vi "FinalizeHWI.vi"(8 "error in (no error)":errorcluster, 10 "Master Device in":refnum<class "Master Device.lvclass">, 11 "Novatech in":refnum<class "Novatech.lvclass">) -> (0 "error out":errorcluster, 2 "Master Device out":refnum<class "Master Device.lvclass">, 3 "Novatech out":refnum<class "Novatech.lvclass">)   [LabVIEW 2013, in "Novatech.lvclass"]
uses:
  Novatech.lvclass
  Master Device/Master Device.lvclass
  Novatech.lvclass/Novatech.ctl
  Novatech 409A.lvlib
panel:
  out "ch2/3 changes?":bool
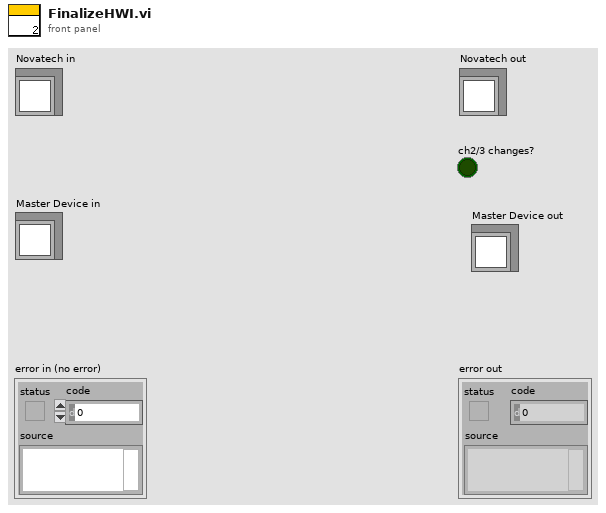
[diagram p1: front panel]
types:
  T1 = cluster{"Triggering":bool[][], "Ramp Info":cluster{"Ramp Index":i32, "Ramp Time":dbl, "Number of Steps":i32}[], "VLIW Array":cluster{"Output Bits":u32, "Data Field":u32, "OP Code":u8, "Delay Count":u64}[]}
  T2 = cluster{"Nova Update List":dbl[][], "2 Freq. [MHz]":dbl, "2 Power [dBm]":u16, "2 phase":u16, "3 Freq. [MHz]":dbl, "3 Power [dBm]":u16, "3 phase":u16}[]
  T3 = cluster{"Freq. [MHz]":dbl[][], "Power [Level]":u16[][], "Phase":u16[][], "2 Freq. [MHz]":dbl, "2 Power [dBm]":u16, "2 phase":u16, "3 Freq. [MHz]":dbl, "3 Power [dBm]":u16, "3 phase":u16}
  T4 = cluster{"Nova Update List":dbl[][], "2 Freq. [MHz]":dbl, "2 Power [dBm]":u16, "2 phase":u16, "3 Freq. [MHz]":dbl, "3 Power [dBm]":u16, "3 phase":u16}
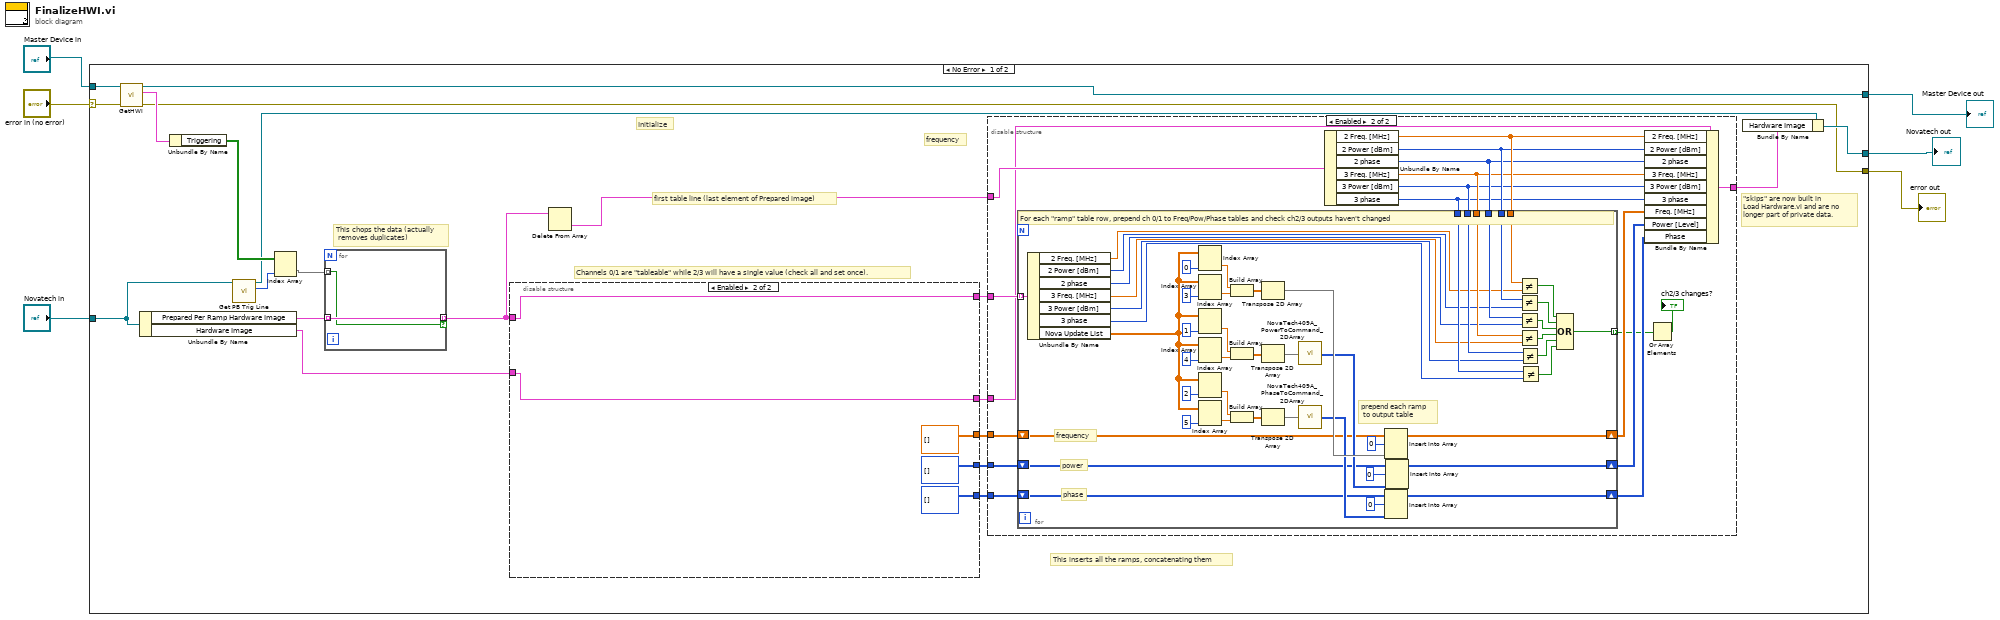
[diagram p0: block diagram]
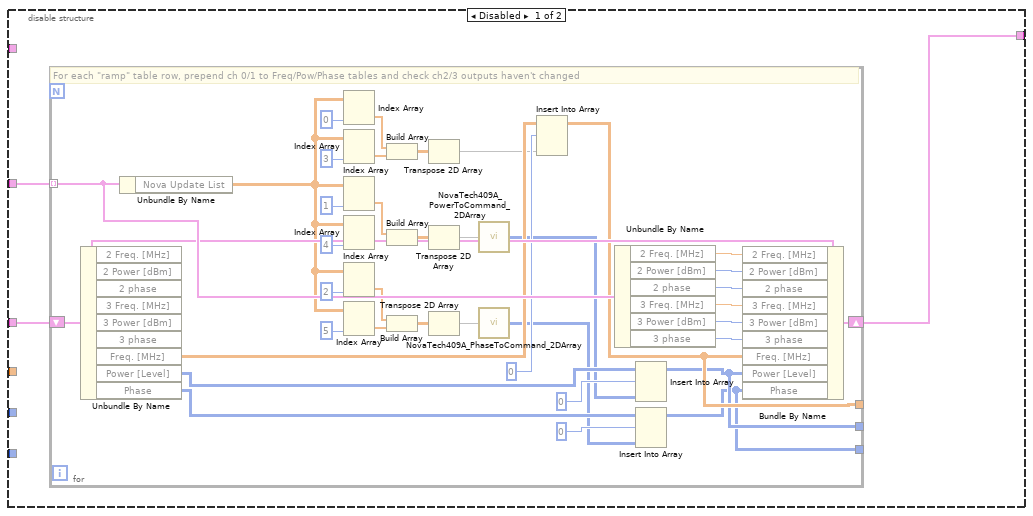
[diagram p2: hidden frame]
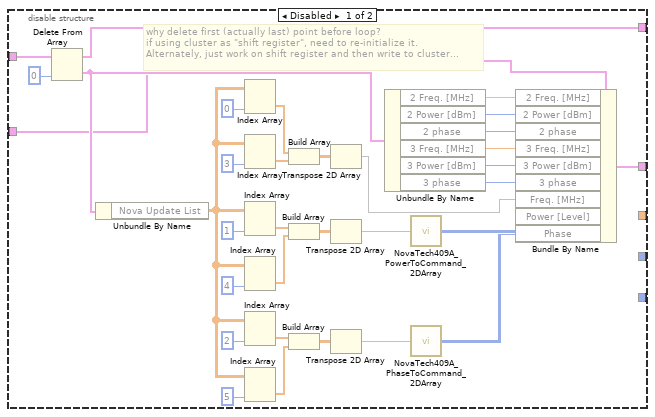
[diagram p3: hidden frame]
diagram:
  n1 = case shown="No Error" "error in (no error)" {
    selector: "error in (no error)" -> [w22 w181]
    tunnel: "Novatech in" -> [w23 w183]
    tunnel: "Master Device in" -> [w26 w182]
    tunnel: [w25 w182] -> w2
    tunnel: [w10 w183] -> w3
    tunnel: [w9 w181] -> w1
    frame No Error {
      # "first table line (last element of Prepared image)"
      # "\"skips\" are now built in \nLoad Hardware.vi and are no \nlonger part of private data."
      # "frequency"
      # "Initialize"
      # "Channels 0/1 are \"tableable\" while 2/3 will have a single value (check all and set once)."
      # "This inserts all the ramps, concatenating them"
      # "This chops the data (actually\n removes duplicates)"
      n2 = call-dynamic "GetHWI.vi"("error in (no error)"=w22, "Master Device in"=w26) -> ("error out"=w9:errorcluster, "Hardware Image"=w24:T1, "Master Device out"=w25:refnum<class "Master Device.lvclass">)  [unwired: 7 in]
      n3 = Unbundle By Name(w23) -> ("Prepared Per Ramp Hardware Image"=w27:T2, "Hardware Image"=w12:T3)
      n4 = Unbundle By Name(w24) -> ("Triggering"=w21:bool[][])
      n5 = call-dynamic "Get PB Trig Line.vi"("Device in"=w23) -> ("PB Trigger Line"=w20:u16, "Device out"=w11:refnum<class "Novatech.lvclass">)  [unwired: 8 in, 1 out]
      n6 = Index Array(array=w21, index (col)=w20) -> (element=w19:bool[])  [unwired: 1 in]
      n7 = for {
        tunnel: w27 -> [w180] mode=indexing
        tunnel: w19 -> [w179] mode=indexing
        tunnel: [w180] -> w8 mode=indexing if=w179
      }
      n8 = disable-structure shown="Enabled" {
        disable-tunnel: w8 -> [w147 w178]
        disable-tunnel: [w144 w177] -> w17
        disable-tunnel: [w143 w178] -> w16
        disable-tunnel: w12 -> [w141 w177]
        disable-tunnel: [_ dbl[][] [] ("Freq. [MHz]")] -> w15
        disable-tunnel: [_ u16[][] [] ("Power [Level]")] -> w14
        disable-tunnel: [_ u16[][] [] ("Phase")] -> w13
        frame Disabled {
          # "why delete first (actually last) point before loop?\nif using cluster as \"shift register\", need to re-initialize it.\nAlternately, just work on shift register and then write to cluster..."
          n9 = Delete From Array(array=w147, index=0) -> (deleted portion=w145:T4, array with subset deleted=w143:T2)  [unwired: 1 in]
          n10 = Unbundle By Name(w145) -> ("Nova Update List"=w155:dbl[][])
          n11 = Index Array(array=w155, index (col)=0) -> (element=w165:dbl[])  [unwired: 1 in]
          n12 = Index Array(array=w155, index (col)=3) -> (element=w164:dbl[])  [unwired: 1 in]
          n13 = Index Array(array=w155, index (col)=1) -> (element=w161:dbl[])  [unwired: 1 in]
          n14 = Index Array(array=w155, index (col)=4) -> (element=w160:dbl[])  [unwired: 1 in]
          n15 = Index Array(array=w155, index (col)=2) -> (element=w157:dbl[])  [unwired: 1 in]
          n16 = Index Array(array=w155, index (col)=5) -> (element=w156:dbl[])  [unwired: 1 in]
          n17 = Build Array(w165, w164) -> (w154:dbl[][])
          n18 = Build Array(w161, w160) -> (w153:dbl[][])
          n19 = Build Array(w157, w156) -> (w152:dbl[][])
          n20 = Transpose 2D Array(2D array=w154) -> (transposed array=w151:dbl[][])
          n21 = Transpose 2D Array(2D array=w153) -> (transposed array=w150:dbl[][])
          n22 = Transpose 2D Array(2D array=w152) -> (transposed array=w148:dbl[][])
          n23 = Unbundle By Name(w145) -> ("2 Freq. [MHz]"=w173:dbl, "2 Power [dBm]"=w172:u16, "2 phase"=w171:u16, "3 Freq. [MHz]"=w170:dbl, "3 Power [dBm]"=w169:u16, "3 phase"=w168:u16)
          n24 = call "NovaTech409A_PowerToCommand_2DArray.vi"("Novatech Power [dBm]"=w150) -> ("Novatech Command"=w149:u16[][])
          n25 = call "NovaTech409A_PhaseToCommand_2DArray.vi"("Novatech Phase [degrees]"=w148) -> ("Novatech Command"=w142:u16[][])
          n26 = Bundle By Name(cluster=w141, "2 Freq. [MHz]"=w173, "2 Power [dBm]"=w172, "2 phase"=w171, "3 Freq. [MHz]"=w170, "3 Power [dBm]"=w169, "3 phase"=w168, "Freq. [MHz]"=w151, "Power [Level]"=w149, "Phase"=w142) -> (w144:T3)
        }
        frame Enabled {
        }
      }
      n27 = Delete From Array(array=w8) -> (deleted portion=w7:T4)  [unwired: 2 in, 1 out]
      n28 = disable-structure shown="Enabled" {
        disable-tunnel: [w33 w86] -> w18
        disable-tunnel: w17 -> [w32 w73]
        disable-tunnel: w16 -> [w31 w90]
        disable-tunnel: w15 -> [_ w89]
        disable-tunnel: w14 -> [_ w88]
        disable-tunnel: w13 -> [_ w87]
        disable-tunnel: w7 -> [_ w82]
        frame Disabled {
          n29 = for {
            tunnel: w31 -> [w72] mode=indexing
            shift-right: [w70] -> w33
            shift-left: w32 -> [w71]
            tunnel: [w69] -> w30
            tunnel: [w68] -> w29
            tunnel: [w34] -> w28
            # "For each \"ramp\" table row, prepend ch 0/1 to Freq/Pow/Phase tables and check ch2/3 outputs haven't changed"
            n30 = Unbundle By Name(w71) -> ("Freq. [MHz]"=w47:dbl[][], "Power [Level]"=w41:u16[][], "Phase"=w40:u16[][])  [unwired: 6 out]
            n31 = Unbundle By Name(w72) -> ("Nova Update List"=w48:dbl[][])
            n32 = Index Array(array=w48, index (col)=0) -> (element=w58:dbl[])  [unwired: 1 in]
            n33 = Index Array(array=w48, index (col)=3) -> (element=w57:dbl[])  [unwired: 1 in]
            n34 = Index Array(array=w48, index (col)=1) -> (element=w54:dbl[])  [unwired: 1 in]
            n35 = Index Array(array=w48, index (col)=4) -> (element=w53:dbl[])  [unwired: 1 in]
            n36 = Index Array(array=w48, index (col)=2) -> (element=w50:dbl[])  [unwired: 1 in]
            n37 = Index Array(array=w48, index (col)=5) -> (element=w49:dbl[])  [unwired: 1 in]
            n38 = Build Array(w58, w57) -> (w46:dbl[][])
            n39 = Build Array(w54, w53) -> (w43:dbl[][])
            n40 = Build Array(w50, w49) -> (w42:dbl[][])
            n41 = Transpose 2D Array(2D array=w46) -> (transposed array=w39:dbl[][])
            n42 = Transpose 2D Array(2D array=w43) -> (transposed array=w38:dbl[][])
            n43 = Transpose 2D Array(2D array=w42) -> (transposed array=w36:dbl[][])
            n44 = call "NovaTech409A_PowerToCommand_2DArray.vi"("Novatech Power [dBm]"=w38) -> ("Novatech Command"=w37:u16[][])
            n45 = call "NovaTech409A_PhaseToCommand_2DArray.vi"("Novatech Phase [degrees]"=w36) -> ("Novatech Command"=w35:u16[][])
            n46 = Insert Into Array(array=w47, index (row)=0, new element=w39) -> (w69:dbl[][])  [unwired: 1 in]
            n47 = Unbundle By Name(w72) -> ("2 Freq. [MHz]"=w66:dbl, "2 Power [dBm]"=w65:u16, "2 phase"=w64:u16, "3 Freq. [MHz]"=w63:dbl, "3 Power [dBm]"=w62:u16, "3 phase"=w61:u16)
            n48 = Insert Into Array(array=w41, index (row)=0, new element=w37) -> (w68:u16[][])  [unwired: 1 in]
            n49 = Insert Into Array(array=w40, index (row)=0, new element=w35) -> (w34:u16[][])  [unwired: 1 in]
            n50 = Bundle By Name(cluster=w71, "2 Freq. [MHz]"=w66, "2 Power [dBm]"=w65, "2 phase"=w64, "3 Freq. [MHz]"=w63, "3 Power [dBm]"=w62, "3 phase"=w61, "Freq. [MHz]"=w69, "Power [Level]"=w68, "Phase"=w34) -> (w70:T3)
          }
        }
        frame Enabled {
          n51 = Unbundle By Name(w82) -> ("2 Freq. [MHz]"=w81:dbl, "2 Power [dBm]"=w80:u16, "2 phase"=w79:u16, "3 Freq. [MHz]"=w78:dbl, "3 Power [dBm]"=w77:u16, "3 phase"=w76:u16)
          n52 = for {
            tunnel: w90 -> [w140] mode=indexing
            shift-right: [w110] -> w85
            shift-left: w89 -> [w115]
            shift-right: [w111] -> w84
            shift-left: w88 -> [w114]
            shift-right: [w112] -> w83
            shift-left: w87 -> [w113]
            tunnel: w81 -> [w103]
            tunnel: w80 -> [w102]
            tunnel: w79 -> [w99]
            tunnel: w78 -> [w98]
            tunnel: w77 -> [w101]
            tunnel: w76 -> [w100]
            tunnel: [w91] -> w75 mode=indexing
            # "prepend each ramp\n to output table"
            # "phase"
            # "power"
            # "frequency"
            # "For each \"ramp\" table row, prepend ch 0/1 to Freq/Pow/Phase tables and check ch2/3 outputs haven't changed"
            n53 = Unbundle By Name(w140) -> ("2 Freq. [MHz]"=w92:dbl, "2 Power [dBm]"=w93:u16, "2 phase"=w94:u16, "3 Freq. [MHz]"=w95:dbl, "3 Power [dBm]"=w96:u16, "3 phase"=w97:u16, "Nova Update List"=w126:dbl[][])
            n54 = Index Array(array=w126, index (col)=0) -> (element=w136:dbl[])  [unwired: 1 in]
            n55 = Index Array(array=w126, index (col)=3) -> (element=w135:dbl[])  [unwired: 1 in]
            n56 = Index Array(array=w126, index (col)=1) -> (element=w132:dbl[])  [unwired: 1 in]
            n57 = Index Array(array=w126, index (col)=4) -> (element=w131:dbl[])  [unwired: 1 in]
            n58 = Index Array(array=w126, index (col)=2) -> (element=w128:dbl[])  [unwired: 1 in]
            n59 = Index Array(array=w126, index (col)=5) -> (element=w127:dbl[])  [unwired: 1 in]
            n60 = Build Array(w136, w135) -> (w125:dbl[][])
            n61 = Build Array(w132, w131) -> (w122:dbl[][])
            n62 = Build Array(w128, w127) -> (w121:dbl[][])
            n63 = Transpose 2D Array(2D array=w125) -> (transposed array=w120:dbl[][])
            n64 = Transpose 2D Array(2D array=w122) -> (transposed array=w119:dbl[][])
            n65 = Transpose 2D Array(2D array=w121) -> (transposed array=w117:dbl[][])
            n66 = call "NovaTech409A_PowerToCommand_2DArray.vi"("Novatech Power [dBm]"=w119) -> ("Novatech Command"=w118:u16[][])
            n67 = call "NovaTech409A_PhaseToCommand_2DArray.vi"("Novatech Phase [degrees]"=w117) -> ("Novatech Command"=w116:u16[][])
            n68 = Insert Into Array(array=w115, index (row)=0, new element=w120) -> (w110:dbl[][])  [unwired: 1 in]
            n69 = Insert Into Array(array=w113, index (row)=0, new element=w116) -> (w112:u16[][])  [unwired: 1 in]
            n70 = Insert Into Array(array=w114, index (row)=0, new element=w118) -> (w111:u16[][])  [unwired: 1 in]
            n71 = Not Equal?(x=w103, y=w92) -> (x != y?=w109:bool)
            n72 = Not Equal?(x=w102, y=w93) -> (x != y?=w108:bool)
            n73 = Not Equal?(x=w99, y=w94) -> (x != y?=w107:bool)
            n74 = Not Equal?(x=w98, y=w95) -> (x != y?=w106:bool)
            n75 = Not Equal?(x=w101, y=w96) -> (x != y?=w104:bool)
            n76 = Not Equal?(x=w100, y=w97) -> (x != y?=w105:bool)
            n77 = Compound Arithmetic op=OR(w109, w108, w107, w106, w104, w105) -> (w91:bool)
          }
          n78 = Bundle By Name(cluster=w73, "2 Freq. [MHz]"=w81, "2 Power [dBm]"=w80, "2 phase"=w79, "3 Freq. [MHz]"=w78, "3 Power [dBm]"=w77, "3 phase"=w76, "Freq. [MHz]"=w85, "Power [Level]"=w84, "Phase"=w83) -> (w86:T3)
          n79 = Or Array Elements(Boolean array=w75) -> (logical OR=→"ch2/3 changes?":bool)
        }
      }
      n80 = Bundle By Name(cluster=w11, "Hardware Image"=w18) -> (w10:refnum<class "Novatech.lvclass">)
    }
    frame Error {
    }
  }
  "error out" <- w1
  "Novatech out" <- w3
  "Master Device out" <- w2
